vi "Main.vi"(11 "Module Admin":refnum<class "Delacor_lib_QMH_Cloneable Module Admin.lvclass">) -> ()   [LabVIEW 2023, in "EL72xxDMC_Drive.lvlib"]
doc: "This template is based off of the Queued Message Handler design pattern and the Queued Message Handler project template that ships with LabVIEW.\n\nThe main difference is that the queue is private to this module and communication between modules is performed via Broadcast and Request events.\n\nRequest events are wrapped in public API methods and are handled in the Event Handling Loop (EHL) of this VI. Any module can register for Broadcast events sent by this module. The EHL generates messages based on user interface actions.\n\nThe Message Handling Loop (MHL) processes messages generated by the EHL, or by other messages. The messages are string values, so new messages can be added easily to the Message Cases case structure in the MHL. Each message cluster can also provide an optional value for Message Data, which is a variant that can be converted to whatever message-specific data is required.\n_____\nBased on DQMH Project Template 7.0.1.1316."
uses:
  EL72xxDMC_Drive.lvlib
  <vilib>/Delacor/Delacor QMH/Libraries/Message Queue_class/Delacor_lib_QMH_Message Queue.lvclass
  Module Data--cluster.ctl
  <vilib>/Utility/miscctls.llb/LVPointTypeDef.ctl
  <vilib>/Delacor/Delacor QMH/Libraries/Message Queue_class/Delacor_lib_QMH_Enqueue Message (Single).vi
  Stop Argument--cluster.ctl
  <vilib>/Delacor/Delacor QMH/Libraries/Cloneable Module Admin_class/Delacor_lib_QMH_Cloneable Module Admin.lvclass
  ConnectToDrive Argument--cluster.ctl
  DisconnectFromDrive Argument--cluster.ctl
  EnableDrive Argument--cluster.ctl
  <userlib>/Beckhoff-LabVIEW-Interface/_DependsOn/Base/TypeResolver/Set TypeResolver.vi
  <userlib>/Beckhoff-LabVIEW-Interface/_DependsOn/Base/Write/Write Sync.vi
  DisableDrive Argument--cluster.ctl
panel:
  out "error out":errorcluster
  out "Status":string
  in  "Simulate EHL Error":bool
  in  "Simulate MHL Error":bool
  # "Other processes communicate with this Module via its Public API (wrappers for its Request Events).\n\nThis Module communicates with other processes via its Broadcast Events.\nAny process that wants to receive these messages can register for this module's Broadcast events."
  # "This template is for the DQMH framework. See the block diagram for more information on how to use this template."
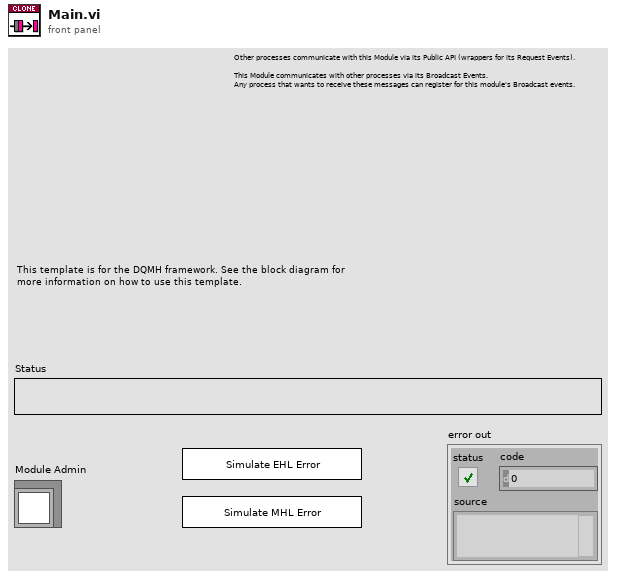
[diagram p1: front panel]
types:
  T1 = typedef "EL72xxDMC_Drive.lvlib/Request Events--cluster.ctl" = cluster{"Stop Module":refnum<user-event>, "Show Panel":refnum<user-event>, "Hide Panel":refnum<user-event>, "Show Diagram":refnum<user-event>, "Get Module Execution Status":refnum<user-event>, "ConnectToDrive":refnum<user-event>, "DisconnectFromDrive":refnum<user-event>, "EnableDrive":refnum<user-event>, "DisableDrive":refnum<user-event>}
  T2 = typedef "EL72xxDMC_Drive.lvlib/Module Data--cluster.ctl" = cluster{"Status":string}
  T3 = enum32{"invalid lock state", "Not Locked", "Locked (No Password)", "Password-protected"}
  T4 = typedef "EL72xxDMC_Drive.lvlib/Stop Argument--cluster.ctl" = cluster{"Module ID":i32, "Origin":string, "Exit via Stop Module Req?":bool, "Wait for Module to stop?":bool}
  T5 = typedef "EL72xxDMC_Drive.lvlib/ConnectToDrive Argument--cluster.ctl" = cluster{"Module ID":i32, "Pathway":string}
  T6 = typedef "EL72xxDMC_Drive.lvlib/DisconnectFromDrive Argument--cluster.ctl" = cluster{"Module ID":i32, "Boolean":bool}
  T7 = typedef "EL72xxDMC_Drive.lvlib/EnableDrive Argument--cluster.ctl" = cluster{"Module ID":i32, "Boolean":bool}
  T8 = typedef "EL72xxDMC_Drive.lvlib/DisableDrive Argument--cluster.ctl" = cluster{"Module ID":i32, "Boolean":bool}
  T9 = typedef "LVPointTypeDef.ctl" = cluster{"Horizontal":i16, "Vertical":i16}
  T10 = enum32{"Invalid", "Standard", "Closed", "Hidden", "Minimized", "Maximized"}
  T11 = cluster{"FeedbackControl":cluster{"Enable latch extern on positive edge":bool, "Set counter":bool, "Enable latch extern on negative edge":bool}, "DriveControl":cluster{"Enable":bool, "Reset":bool}, "PositioningControl":cluster{"Execute":bool, "Emergency stop":bool}, "Set counter value":i32, "Target position":i32, "Target velocity":i16, "Start type":u16, "Target acceleration":u16, "Target deceleration":u16}
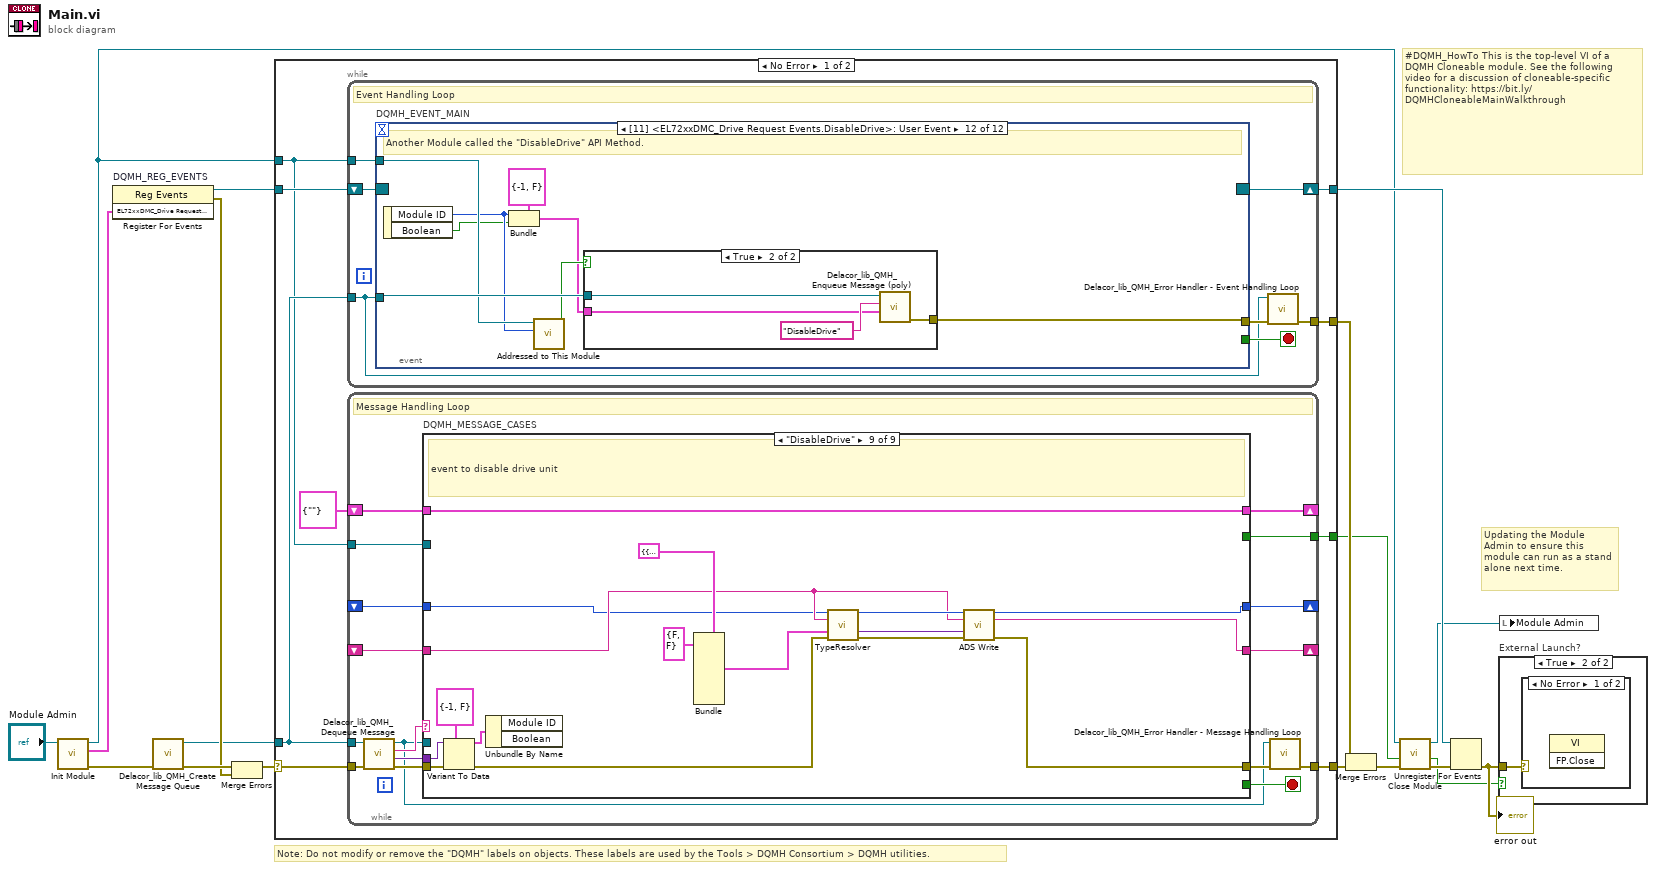
[diagram p0: block diagram]
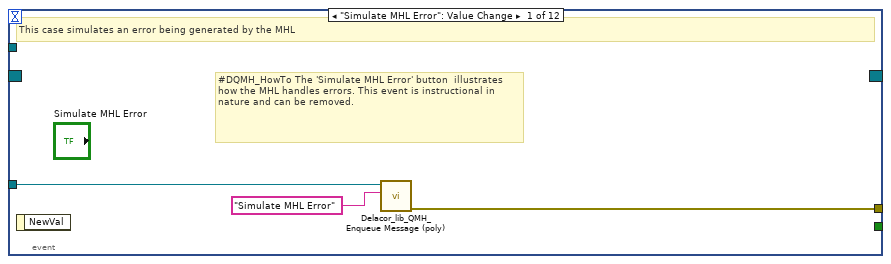
[diagram p2: hidden frame]
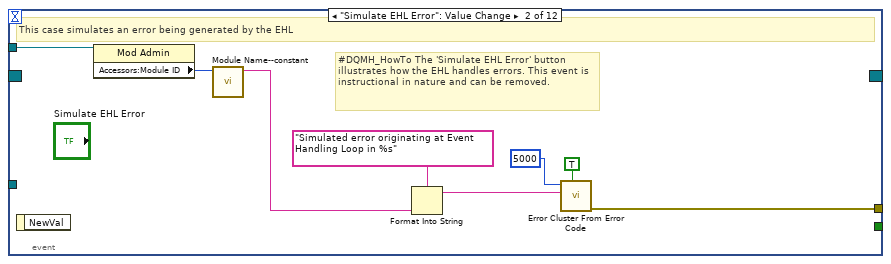
[diagram p3: hidden frame]
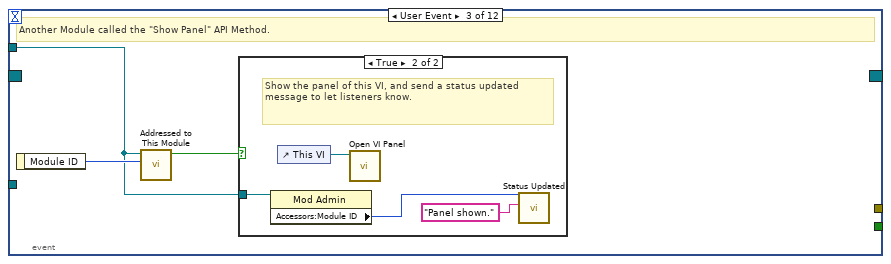
[diagram p4: hidden frame]
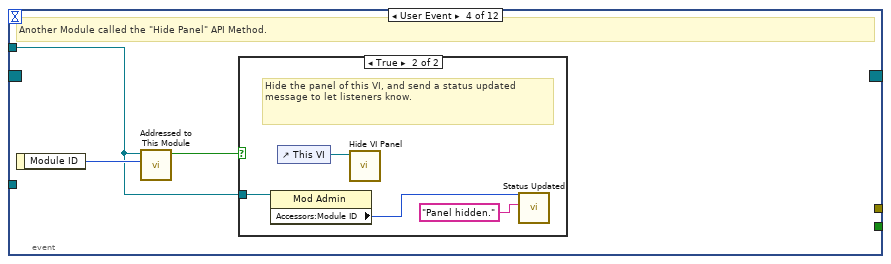
[diagram p6: hidden frame]
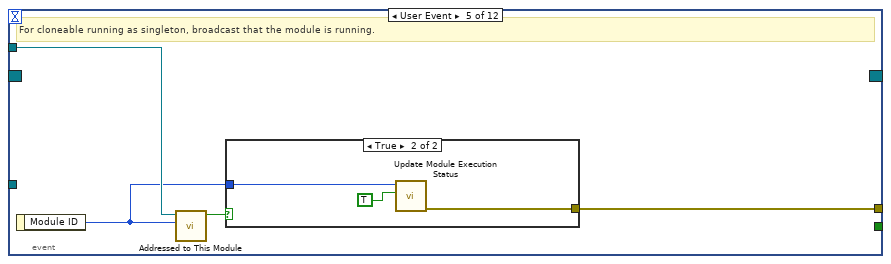
[diagram p8: hidden frame]
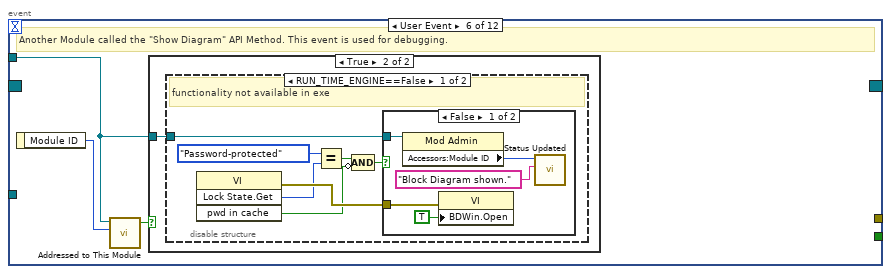
[diagram p10: hidden frame]
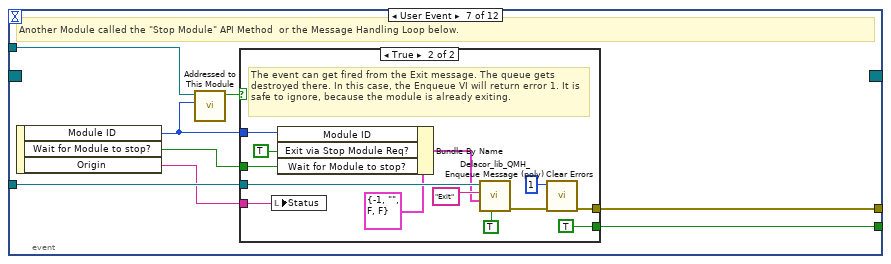
[diagram p14: hidden frame]
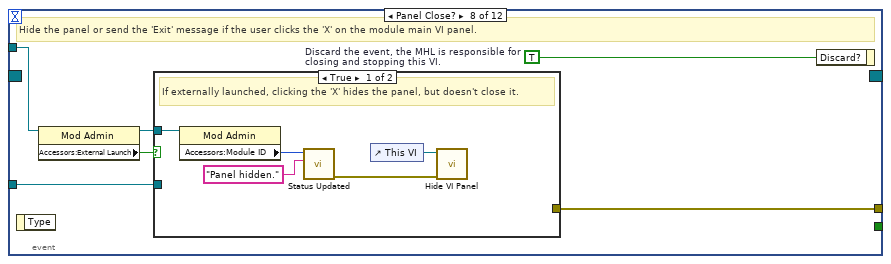
[diagram p16: hidden frame]
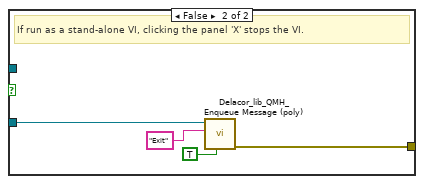
[diagram p17: hidden frame]
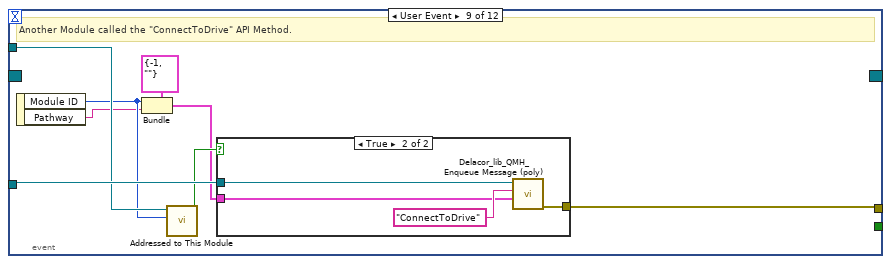
[diagram p18: hidden frame]
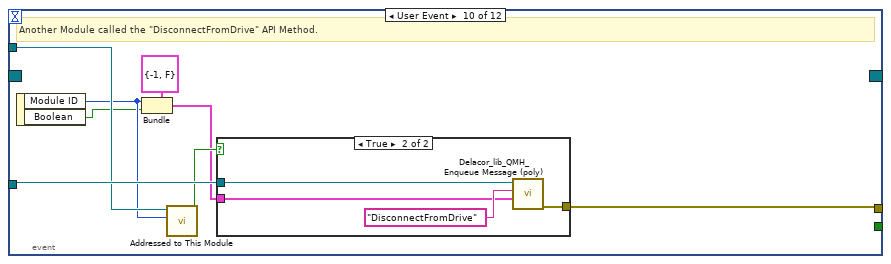
[diagram p20: hidden frame]
diagram:
  # "#DQMH_HowTo This is the top-level VI of a DQMH Cloneable module. See the following video for a discussion of cloneable-specific functionality: https://bit.ly/DQMHCloneableMainWalkthrough"
  # "Note: Do not modify or remove the \"DQMH\" labels on objects. These labels are used by the Tools > DQMH Consortium > DQMH utilities."
  # "Updating the Module Admin to ensure this module can run as a stand alone next time."
  n1 = call "Init Module.vi"("Cloneable Module Admin in"="Module Admin") -> ("error out"=w15:errorcluster, "EL72xxDMC_Drive Request Events"=w7:T1, "Cloneable Module Admin out"=w4:refnum<class "Delacor_lib_QMH_Cloneable Module Admin.lvclass">)  [unwired: 8 in]
  n2 = register-events "DQMH_REG_EVENTS"(w7) -> (reference out=w8:refnum<event-registration>, error out=w10:errorcluster)  [unwired: 2 in]
  n3 = call <vilib>:"Delacor_lib_QMH_Create Message Queue.vi"("error in"=w15) -> ("error out"=w12:errorcluster, "Message Queue"=w6:refnum<class "Delacor_lib_QMH_Message Queue.lvclass">)  [unwired: 9 in]
  n4 = Merge Errors(w12, w10) -> (w11:errorcluster)
  n5 = case shown="No Error" w11 {
    selector: w11 -> [w25 w338]
    tunnel: [w27 w337] -> w16
    tunnel: [w24 w336] -> w9
    tunnel: w8 -> [w22 w336]
    tunnel: w6 -> [w21 w329]
    tunnel: [w26 _] -> w17
    tunnel: w4 -> [w20 w332]
    tunnel: [w19 _] -> w2
    frame No Error {
      n6 = while {
        tunnel: w21 -> [w28]
        shift-right: [w31] -> w24
        shift-left: w22 -> [w32]
        tunnel: [w33] -> w26
        tunnel: w20 -> [w29]
        stop <- w30 stop-if-true
        # "Event Handling Loop"
        n7 = event "DQMH_EVENT_MAIN" shown="[11] <EL72xxDMC_Drive Request Events.DisableDrive>: User Event" {
          selector: w32 -> [_ _ _ _ _ _ _ _ _ _ _ _]
          dyn-events: [_ _ _ _ _ _ _ _ _ _ _ _] -> w31
          timeout: _ -> [_ _ _ _ _ _ _ _ _ _ _ _]
          tunnel: [_ _ _ _ _ _ w86 _ _ _ _ _] -> w30
          tunnel: w28 -> [w36 _ _ _ _ _ w89 w106 w126 w138 w150 w162]
          tunnel: [w37 w45 _ _ w63 _ w90 w109 w119 w131 w143 w155] -> w34
          tunnel: w29 -> [_ w44 w46 w53 w61 w67 w88 w107 w124 w136 w148 w160]
          event "Simulate MHL Error": Value Change {
            # "#DQMH_HowTo The 'Simulate MHL Error' button  illustrates how the MHL handles errors. This event is instructional in nature and can be removed."
            # "This case simulates an error being generated by the MHL"
            n8 = event-data() -> ()  [unwired: 1 in, 1 out]
            n9 = call-poly <vilib>:"Delacor_lib_QMH_Enqueue Message (poly).vi"("Message"="Simulate MHL Error", "Message Queue in"=w36) -> ("error out"=w37:errorcluster)  [unwired: 8 in, 1 out]
          }
          event "Simulate EHL Error": Value Change {
            # "#DQMH_HowTo The 'Simulate EHL Error' button  illustrates how the EHL handles errors. This event is instructional in nature and can be removed."
            # "This case simulates an error being generated by the EHL"
            n10 = event-data() -> ()  [unwired: 1 in, 1 out]
            n11 = property on="Property Node" class="Mod Admin"(reference=w44) -> ("Accessors:Module ID"=w43:i32)  [unwired: 1 in, 2 out]
            n12 = call "Module Name--constant.vi"("Module ID"=w43) -> ("Module Name"=w38:string)  [unwired: 10 in]
            n13 = Format Into String(format string="Simulated error originating at Event Handling Loop in %s", w38) -> (resulting string=w41:string)  [unwired: 2 in, 1 out]
            n14 = call <vilib>:"Error Cluster From Error Code.vi"("show call chain? (False)"=TRUE, "error message (\"\")"=w41, "error code (0)"=5000) -> ("error out"=w45:errorcluster)  [unwired: 6 in]
          }
          event User Event {
            # "Another Module called the \"Show Panel\" API Method."
            n15 = event-data() -> ("Module ID"=w47:i32)  [unwired: 1 in]
            n16 = call "Addressed to This Module.vi"("Module ID from Argument"=w47, "Module Admin"=w46) -> ("Addressed to this instance?"=w48:bool)  [unwired: 8 in, 1 out]
            n17 = case shown="True" w48 {
              tunnel: w46 -> [_ w50]
              frame False {
              }
              frame True {
                # "Show the panel of this VI, and send a status updated message to let listeners know."
                n18 = property on="Property Node" class="Mod Admin"(reference=w50) -> ("Accessors:Module ID"=w49:i32)  [unwired: 1 in, 2 out]
                n19 = control-ref of="This VI"() -> (w52:refnum<vi>)
                n20 = call "Open VI Panel.vi"("VI"=w52) -> ()  [unwired: 10 in, 1 out]
                n21 = call "Status Updated.vi"("Status"="Panel shown." ("format string"), "Module ID"=w49) -> ()  [unwired: 9 in, 1 out]
              }
            }
          }
          event User Event {
            # "Another Module called the \"Hide Panel\" API Method."
            n22 = event-data() -> ("Module ID"=w54:i32)  [unwired: 1 in]
            n23 = call "Addressed to This Module.vi"("Module ID from Argument"=w54, "Module Admin"=w53) -> ("Addressed to this instance?"=w55:bool)  [unwired: 8 in, 1 out]
            n24 = case shown="True" w55 {
              tunnel: w53 -> [_ w57]
              frame False {
              }
              frame True {
                # "Hide the panel of this VI, and send a status updated message to let listeners know."
                n25 = property on="Property Node" class="Mod Admin"(reference=w57) -> ("Accessors:Module ID"=w56:i32)  [unwired: 1 in, 2 out]
                n26 = control-ref of="This VI"() -> (w59:refnum<vi>)
                n27 = call "Hide VI Panel.vi"("VI"=w59) -> ()  [unwired: 10 in, 1 out]
                n28 = call "Status Updated.vi"("Status"="Panel hidden." ("format string"), "Module ID"=w56) -> ()  [unwired: 9 in, 1 out]
              }
            }
          }
          event User Event {
            # "For cloneable running as singleton, broadcast that the module is running."
            n29 = event-data() -> ("Module ID"=w60:i32)  [unwired: 1 in]
            n30 = call "Addressed to This Module.vi"("Module ID from Argument"=w60, "Module Admin"=w61) -> ("Addressed to this instance?"=w62:bool)  [unwired: 8 in, 1 out]
            n31 = case shown="True" w62 {
              tunnel: [_ w66] -> w63
              tunnel: w60 -> [_ w65]
              frame False {
              }
              frame True {
                n32 = call "Update Module Execution Status.vi"("Running?"=TRUE, "Module ID"=w65) -> ("error out"=w66:errorcluster)  [unwired: 9 in]
              }
            }
          }
          event User Event {
            # "Another Module called the \"Show Diagram\" API Method. This event is used for debugging."
            n33 = event-data() -> ("Module ID"=w68:i32)  [unwired: 1 in]
            n34 = call "Addressed to This Module.vi"("Module ID from Argument"=w68, "Module Admin"=w67) -> ("Addressed to this instance?"=w69:bool)  [unwired: 8 in, 1 out]
            n35 = case shown="True" w69 {
              tunnel: w67 -> [_ w70]
              frame False {
              }
              frame True {
                n36 = disable-structure shown="RUN_TIME_ENGINE==False" {
                  disable-tunnel: w70 -> [w71 _]
                  frame condition #0 (active) {
                    # "functionality not available in exe"
                    n37 = invoke on="Invoke Node" class="VI" method="Lock State.Get"() -> (error out=w77:errorcluster, "Get Lock State"=w76:T3, "pwd in cache"=w73:bool)  [unwired: 4 in, 1 out]
                    n38 = Equal?(x=T3."Password-protected", y=w76) -> (x = y?=w74:bool)
                    n39 = Compound Arithmetic op=AND(w74, invert w73) -> (w72:bool)
                    n40 = case shown="False" w72 {
                      tunnel: w77 -> [w82 _]
                      tunnel: w71 -> [w79 _]
                      frame False {
                        n41 = property on="Property Node" class="Mod Admin"(reference=w79) -> ("Accessors:Module ID"=w78:i32)  [unwired: 1 in, 2 out]
                        n42 = property on="Property Node" class="VI"(error in=w82, "BDWin.Open"=TRUE ("Block Diagram Window:Open")) -> ()  [unwired: 1 in, 2 out]
                        n43 = call "Status Updated.vi"("Status"="Block Diagram shown." ("format string"), "Module ID"=w78) -> ()  [unwired: 9 in, 1 out]
                      }
                      frame True {
                        # "Password-protected VI, and the password is not in the cache. Do not show the diagram."
                      }
                    }
                  }
                  frame condition #1 {
                  }
                }
              }
            }
          }
          event User Event {
            # "Another Module called the \"Stop Module\" API Method  or the Message Handling Loop below."
            n44 = event-data() -> ("Module ID"=w84:i32, "Wait for Module to stop?"=w85:bool, "Origin"=w83:string)  [unwired: 1 in]
            n45 = call "Addressed to This Module.vi"("Module ID from Argument"=w84, "Module Admin"=w88) -> ("Addressed to this instance?"=w87:bool)  [unwired: 8 in, 1 out]
            n46 = case shown="True" w87 {
              tunnel: [_ w102] -> w90
              tunnel: w89 -> [_ w98]
              tunnel: [_ TRUE] -> w86
              tunnel: w85 -> [_ w93]
              tunnel: w84 -> [_ w95]
              tunnel: w83 -> [_ w91]
              frame False {
              }
              frame True {
                # "The event can get fired from the Exit message. The queue gets destroyed there. In this case, the Enqueue VI will return error 1. It is safe to ignore, because the module is already exiting."
                n47 = local write "Status"(w91) -> ()
                n48 = Bundle By Name(cluster=T4 {"Module ID"=-1, "Origin"="", "Exit via Stop Module Req?"=FALSE, "Wait for Module to stop?"=FALSE} ("Stop Argument"), "Module ID"=w95, "Exit via Stop Module Req?"=TRUE, "Wait for Module to stop?"=w93) -> (w92:T4)
                n49 = call-poly <vilib>:"Delacor_lib_QMH_Enqueue Message (poly).vi"("Priority Message? (F)"=TRUE, "Message Data"=w92, "Message"="Exit", "Message Queue in"=w98) -> ("error out"=w103:errorcluster)  [unwired: 6 in, 1 out]
                n50 = call <vilib>:"Clear Errors.vi"("error in (no error)"=w103, "specific error code to clear (0: all)"=1) -> ("error out"=w102:errorcluster)  [unwired: 4 in, 1 out]
              }
            }
          }
          event Panel Close? {
            w108 = TRUE  # Discard the event, the MHL is responsible for closing and stopping this VI.
            # "Hide the panel or send the 'Exit' message if the user clicks the 'X' on the module main VI panel."
            n51 = event-data() -> ()  [unwired: 1 in, 1 out]
            n52 = property on="Property Node" class="Mod Admin"(reference=w107) -> (reference out=w104:refnum<class "Delacor_lib_QMH_Cloneable Module Admin.lvclass">, "Accessors:External Launch"=w105:bool)  [unwired: 1 in, 1 out]
            n53 = case shown="True" w105 {
              tunnel: w106 -> [_ w117]
              tunnel: [_ w118] -> w109
              tunnel: w104 -> [w112 _]
              frame True {
                # "If externally launched, clicking the 'X' hides the panel, but doesn't close it."
                n54 = property on="Property Node" class="Mod Admin"(reference=w112) -> ("Accessors:Module ID"=w111:i32)  [unwired: 1 in, 2 out]
                n55 = call "Status Updated.vi"("Status"="Panel hidden." ("format string"), "Module ID"=w111) -> ("error out"=w110:errorcluster)  [unwired: 9 in]
                n56 = control-ref of="This VI"() -> (w114:refnum<vi>)
                n57 = call "Hide VI Panel.vi"("error in"=w110, "VI"=w114) -> ()  [unwired: 9 in, 1 out]
              }
              frame False {
                # "If run as a stand-alone VI, clicking the panel 'X' stops the VI."
                n58 = call-poly <vilib>:"Delacor_lib_QMH_Enqueue Message (poly).vi"("Priority Message? (F)"=TRUE, "Message"="Exit", "Message Queue in"=w117) -> ("error out"=w118:errorcluster)  [unwired: 7 in, 1 out]
              }
            }
            n59 = event-data ("Event Filter Node")("Discard?"=w108) -> ()  [unwired: 1 in, 1 out]
          }
          event User Event {
            # "Another Module called the \"ConnectToDrive\" API Method."
            n60 = event-data() -> ("Module ID"=w121:i32, "Pathway"=w120:string)  [unwired: 1 in]
            n61 = Bundle(cluster=T5 {"Module ID"=-1, "Pathway"=""} ("ConnectToDrive Argument"), "Module ID"=w121, "Pathway"=w120) -> (w122:T5)
            n62 = call "Addressed to This Module.vi"("Module ID from Argument"=w121, "Module Admin"=w124) -> ("Addressed to this instance?"=w125:bool)  [unwired: 8 in, 1 out]
            n63 = case shown="True" w125 {
              tunnel: w126 -> [_ w130]
              tunnel: w122 -> [_ w128]
              tunnel: [_ w127] -> w119
              frame False {
              }
              frame True {
                n64 = call-poly <vilib>:"Delacor_lib_QMH_Enqueue Message (poly).vi"("Message Data"=w128, "Message"="ConnectToDrive", "Message Queue in"=w130) -> ("error out"=w127:errorcluster)  [unwired: 7 in, 1 out]
              }
            }
          }
          event User Event {
            # "Another Module called the \"DisconnectFromDrive\" API Method."
            n65 = event-data() -> ("Module ID"=w133:i32, "Boolean"=w132:bool)  [unwired: 1 in]
            n66 = Bundle(cluster=T6 {"Module ID"=-1, "Boolean"=FALSE} ("DisconnectFromDrive Argument"), "Module ID"=w133, "Boolean"=w132) -> (w134:T6)
            n67 = call "Addressed to This Module.vi"("Module ID from Argument"=w133, "Module Admin"=w136) -> ("Addressed to this instance?"=w137:bool)  [unwired: 8 in, 1 out]
            n68 = case shown="True" w137 {
              tunnel: w138 -> [_ w142]
              tunnel: w134 -> [_ w140]
              tunnel: [_ w139] -> w131
              frame False {
              }
              frame True {
                n69 = call-poly <vilib>:"Delacor_lib_QMH_Enqueue Message (poly).vi"("Message Data"=w140, "Message"="DisconnectFromDrive", "Message Queue in"=w142) -> ("error out"=w139:errorcluster)  [unwired: 7 in, 1 out]
              }
            }
          }
          event User Event {
            # "Another Module called the \"EnableDrive\" API Method."
            n70 = event-data() -> ("Module ID"=w145:i32, "Boolean"=w144:bool)  [unwired: 1 in]
            n71 = Bundle(cluster=T7 {"Module ID"=-1, "Boolean"=FALSE} ("EnableDrive Argument"), "Module ID"=w145, "Boolean"=w144) -> (w146:T7)
            n72 = call "Addressed to This Module.vi"("Module ID from Argument"=w145, "Module Admin"=w148) -> ("Addressed to this instance?"=w149:bool)  [unwired: 8 in, 1 out]
            n73 = case shown="True" w149 {
              tunnel: w150 -> [_ w154]
              tunnel: w146 -> [_ w152]
              tunnel: [_ w151] -> w143
              frame False {
              }
              frame True {
                n74 = call-poly <vilib>:"Delacor_lib_QMH_Enqueue Message (poly).vi"("Message Data"=w152, "Message"="EnableDrive", "Message Queue in"=w154) -> ("error out"=w151:errorcluster)  [unwired: 7 in, 1 out]
              }
            }
          }
          event User Event {
            # "Another Module called the \"DisableDrive\" API Method."
            n75 = event-data() -> ("Module ID"=w157:i32, "Boolean"=w156:bool)  [unwired: 1 in]
            n76 = Bundle(cluster=T8 {"Module ID"=-1, "Boolean"=FALSE} ("DisableDrive Argument"), "Module ID"=w157, "Boolean"=w156) -> (w158:T8)
            n77 = call "Addressed to This Module.vi"("Module ID from Argument"=w157, "Module Admin"=w160) -> ("Addressed to this instance?"=w161:bool)  [unwired: 8 in, 1 out]
            n78 = case shown="True" w161 {
              tunnel: w162 -> [_ w166]
              tunnel: w158 -> [_ w164]
              tunnel: [_ w163] -> w155
              frame False {
              }
              frame True {
                n79 = call-poly <vilib>:"Delacor_lib_QMH_Enqueue Message (poly).vi"("Message Data"=w164, "Message"="DisableDrive", "Message Queue in"=w166) -> ("error out"=w163:errorcluster)  [unwired: 7 in, 1 out]
              }
            }
          }
        }
        n80 = call-dynamic "Delacor_lib_QMH_Error Handler - Event Handling Loop.vi"("error in"=w34, "Message Queue in"=w28) -> ("dup error in"=w33:errorcluster)  [unwired: 8 in, 1 out]
      }
      n81 = while {
        tunnel: w21 -> [w171]
        shift-right: [w178] -> _
        shift-left: T2 {"Status"=""} ("Data Cluster") -> [w179]
        tunnel: w25 -> [w182]
        tunnel: [w180] -> w27
        tunnel: w20 -> [w173]
        tunnel: [w172] -> w19
        shift-right: [w170] -> _
        shift-left: _ -> [w167]
        shift-right: [w169] -> _
        shift-left: _ -> [w168]
        stop <- w177 stop-if-true
        # "Message Handling Loop"
        n82 = call-dynamic "Delacor_lib_QMH_Dequeue Message.vi"("error in"=w182, "Message Queue in"=w171) -> ("error out"=w181:errorcluster, "Message Data"=w175:variant, "Message"=w176:string, "Message Queue out"=w174:refnum<class "Delacor_lib_QMH_Message Queue.lvclass">)  [unwired: 6 in]
        n83 = case "DQMH_MESSAGE_CASES" shown="\"DisableDrive\"" w176 {
          selector: w176 -> [_ _ _ _ _ w274 _ _ _]
          tunnel: w174 -> [_ _ w223 _ w264 _ _ _ _]
          tunnel: w181 -> [w204 w218 w232 w251 w270 w283 w294 w311 w328]
          tunnel: [w202 w211 w228 w250 w265 w284 w287 w302 w312] -> w183
          tunnel: w179 -> [w195 w217 w227 w248 w263 w281 w293 w310 w327]
          tunnel: [w194 w217 w227 w248 w263 w281 w293 w310 w327] -> w178
          tunnel: [_ _ _ _ w262 _ _ _ _] -> w177
          tunnel: w175 -> [_ w216 w226 _ w260 _ w292 w309 w326]
          tunnel: w173 -> [w189 _ w225 w246 w255 w280 _ _ _]
          tunnel: [_ _ _ _ w258 _ _ _ _] -> w172
          tunnel: [u32 0 ("Handle") w210 u32 0 ("Handle") u32 0 ("Handle") u32 0 ("Handle") w271 u32 0 ("Handle") w299 w315] -> w170
          tunnel: ["" ("ReadGrpSymbols") w207 "" ("ReadGrpSymbols") "" ("ReadGrpSymbols") "" ("ReadGrpSymbols") w272 "" ("ReadGrpSymbols") w298 w314] -> w169
          tunnel: w168 -> [_ _ _ _ _ w272 _ w300 w317]
          tunnel: w167 -> [_ _ _ _ _ w271 w289 w306 w316]
          frame "Initialize" {
            w186 = "Initial Message" ("Initial Message")
            # "#CodeNeeded - Initialize the appearance of the front panel."
            # "#CodeNeeded - Initialize your state data here."
            # "Initialize - Any operation that needs to be done before the module can receive messages. Synchronize Caller Events.vi will inform Start Module.vi that the module has launched and is ready to receive messages. Module Did Init.vi will broadcast that the module initialized."
            n84 = call "Synchronize Caller Events.vi"("error in"=w204, "Module Admin"=w189) -> ("error out"=w203:errorcluster, "Module Admin out"=w188:refnum<class "Delacor_lib_QMH_Cloneable Module Admin.lvclass">)  [unwired: 8 in]
            n85 = property on="Property Node" class="Mod Admin"(reference=w188) -> ("Accessors:Module ID"=w191:i32, "Accessors:External Launch"=w190:bool)  [unwired: 1 in, 2 out]
            n86 = call "Module Name--constant.vi"("Module ID"=w191) -> ("Module Name"=w199:string)  [unwired: 10 in]
            n87 = property on="Property Node" class="VI"("Front Panel.Title"=w199) -> (reference out=w201:refnum<vi>, error out=w206:errorcluster)  [unwired: 2 in]
            n88 = Select(t=T10."Hidden" ("State"), s=w190, f=T10."Standard" ("State")) -> (s? t:f=w196:T10)
            n89 = invoke on="Invoke Node" class="VI" method="FP.Open"(reference=w201, error in=w206, "State"=w196) -> (reference out=w200:refnum<vi>, error out=w205:errorcluster)  [unwired: 2 in, 3 out]
            n90 = call "Module Name--constant.vi"("Module ID"=w191) -> ("Module Name"=w192:string)  [unwired: 10 in]
            n91 = Bundle By Name(cluster=w195, "Status"=w186) -> (w194:T2)
            n92 = invoke on="Invoke Node" class="VI" method="FP.Center"(reference=w200, error in=w205) -> ()  [unwired: 1 in, 3 out]
            n93 = property on="Pane" class="Pane"("Origin"=T9 {"Horizontal"=0, "Vertical"=0}) -> ()  [unwired: 2 in, 2 out]
            n94 = call "Module Did Init.vi"("error in"=w203, "Initialized?"=TRUE, "Origin"=w192, "Module ID"=w191) -> ("error out"=w202:errorcluster)  [unwired: 7 in]
            "Status" <- w186
          }
          frame "ConnectToDrive" {
            # "event to create a connection to a drive terminal"
            n95 = Variant To Data(error in=w218, type=T5 {"Module ID"=-1, "Pathway"=""} ("ConnectToDrive Argument"), Variant=w216) -> (data=w214:T5, error out=w212:errorcluster)
            n96 = Unbundle By Name(w214) -> ("Pathway"=w213:string)  [unwired: 1 out]
            n97 = call <userlib>:"Init.vi"("XMLDescription"=w213, "error in (no error)"=w212) -> ("Handle"=w210:u32, "WriteGrpSymbols"=w209:string[], "error out"=w211:errorcluster)  [unwired: 9 in, 2 out]
            n98 = Index Array(array=w209, index=0) -> (element=w207:string)
          }
          frame "Error" {
            # "#CodeRecommended - If the module is running in standalone mode (External Launch = FALSE), this code will pop up an error dialog and call the 'Exit' message if an error occurs. Add more fine-grained error management here."
            # "Error - Check the error message data and respond accordingly. This message is sent by the \"Error Handler\" VIs at the end of each loop in this application."
            n99 = property on="Property Node" class="Mod Admin"(reference=w225) -> ("Accessors:External Launch"=w224:bool, "Accessors:Module ID"=w222:i32)  [unwired: 1 in, 2 out]
            n100 = Variant To Data(error in=w232, type=errorcluster {"status"=FALSE, "code"=0, "source"=""} ("error constant"), Variant=w226) -> (data=w221:errorcluster, error out=w230:errorcluster)
            n101 = local write "error out"(w221) -> ()
            n102 = call "Error Reported.vi"("Error"=w221, "Module ID"=w222) -> ()  [unwired: 9 in, 1 out]
            n103 = case shown="False" w224 {
              tunnel: [w237 _] -> w229
              tunnel: w223 -> [w235 _]
              tunnel: w221 -> [w236 _]
              frame False {
                n104 = disable-structure shown="Default" {
                  disable-tunnel: w236 -> [w238 _]
                  frame condition #0 (active) {
                    # "If the module is running standalone, then pop up an error dialog and call the \"Exit\" message."
                    n105 = call <vilib>:"Simple Error Handler.vi"("error in (no error)"=w238) -> ()  [unwired: 4 in, 5 out]
                  }
                  frame condition #1 {
                    # "To prevent the Simple Error Handler VI from being loaded (e.g. when deploying to a Real-Time target), add the Conditional Disable Symbol \"DQMH_Disable_SEH\" to your project and set it to TRUE."
                  }
                }
                n106 = call-poly <vilib>:"Delacor_lib_QMH_Enqueue Message (poly).vi"("Priority Message? (F)"=TRUE, "Message"="Exit", "Message Queue in"=w235) -> ("error out"=w237:errorcluster)  [unwired: 7 in, 1 out]
              }
              frame True {
                # "If the module was launched externally, calling the Error Reported broadcast VI is the only action performed by the \"Error\" message. The module's caller can then process the error appropriately."
              }
            }
            n107 = Merge Errors(w230, w229) -> (w228:errorcluster)
          }
          frame "Simulate MHL Error" {
            # "#DQMH_HowTo The 'Simulate MHL Error' button  illustrates how the MHL handles errors. This event is instructional in nature and can be removed."
            # "Simulate an error occurring at the MHL"
            n108 = property on="Property Node" class="Mod Admin"(reference=w246) -> ("Accessors:Module ID"=w247:i32)  [unwired: 1 in, 2 out]
            n109 = call "Module Name--constant.vi"("Module ID"=w247) -> ("Module Name"=w242:string)  [unwired: 10 in]
            n110 = Format Into String(format string="Simulated error originating at Message Handling Loop in %s", w242) -> (resulting string=w243:string)  [unwired: 2 in, 1 out]
            n111 = call <vilib>:"Error Cluster From Error Code.vi"("show call chain? (False)"=TRUE, "error message (\"\")"=w243, "error code (0)"=5001) -> ("error out"=w249:errorcluster)  [unwired: 6 in]
            n112 = Merge Errors(w251, w249) -> (w250:errorcluster)
          }
          frame "Exit" {
            w261 = 91  # 91: not all Exit messages will have an argument
            w262 = TRUE  # Stop the VI
            # "Release the message queue reference"
            # "#CodeNeeded - Add any required cleanup code here."
            # "Exit - Exit the application."
            n113 = Variant To Data(error in=w270, type=T4 {"Module ID"=-1, "Origin"="", "Exit via Stop Module Req?"=FALSE, "Wait for Module to stop?"=FALSE} ("Stop Argument"), Variant=w260) -> (data=w257:T4, error out=w266:errorcluster)
            n114 = call <vilib>:"Clear Errors.vi"("error in (no error)"=w266, "specific error code to clear (0: all)"=w261) -> ("error out"=w269:errorcluster)  [unwired: 4 in, 1 out]
            n115 = property on="Property Node" class="Mod Admin"(reference=w255) -> ("Accessors:Module ID"=w254:i32)  [unwired: 1 in, 2 out]
            n116 = control-ref of="This VI"() -> (w256:refnum<vi>)
            n117 = call-dynamic "Delacor_lib_QMH_Release Message Queue.vi"("error in"=w269, "Message Queue"=w264) -> ("error out"=w268:errorcluster)  [unwired: 9 in]
            n118 = call "Handle Exit.vi"("Stop Argument"=w257, "Module Admin in"=w255, "VI reference"=w256) -> ("error out"=w267:errorcluster, "Wait for Stop?"=w258:bool)  [unwired: 7 in]
            n119 = Merge Errors(w268, w267) -> (w265:errorcluster)
            n120 = call "Error Reported.vi"("Error"=w265, "Module ID"=w254) -> ()  [unwired: 9 in, 1 out]
          }
          frame Default {
            # "'Default' case only runs if there is a message that isn't defined in any of the other cases.  Output a programming error."
            n121 = property on="Property Node" class="Mod Admin"(reference=w280) -> ("Accessors:Module ID"=w279:i32)  [unwired: 1 in, 2 out]
            n122 = call "Module Name--constant.vi"("Module ID"=w279) -> ("Module Name"=w273:string)  [unwired: 10 in]
            n123 = Format Into String(format string="The invalid message string \"%s\" was received in the Message Handling Loop for module \"%s\".", w274, w273) -> (resulting string=w276:string)  [unwired: 2 in, 1 out]
            n124 = call <vilib>:"Error Cluster From Error Code.vi"("show call chain? (False)"=TRUE, "error message (\"\")"=w276, "error code (0)"=1) -> ("error out"=w282:errorcluster)  [unwired: 6 in]
            n125 = Merge Errors(w283, w282) -> (w284:errorcluster)
          }
          frame "DisconnectFromDrive" {
            # "event to disconnect from a drive temrinal"
            n126 = Variant To Data(error in=w294, type=T6 {"Module ID"=-1, "Boolean"=FALSE} ("DisconnectFromDrive Argument"), Variant=w292) -> (data=w290:T6, error out=w288:errorcluster)
            n127 = Unbundle By Name(w290) -> ()  [unwired: 2 out]
            n128 = call <userlib>:"Release.vi"("Handle"=w289, "error in (no error)"=w288) -> ("error out"=w287:errorcluster)  [unwired: 13 in]
          }
          frame "EnableDrive" {
            n129 = Variant To Data(error in=w311, type=T7 {"Module ID"=-1, "Boolean"=FALSE} ("EnableDrive Argument"), Variant=w309) -> (data=w307:T7, error out=w305:errorcluster)
            n130 = Unbundle By Name(w307) -> ()  [unwired: 2 out]
            n131 = Bundle(cluster=T11 {"FeedbackControl"={"Enable latch extern on positive edge"=FALSE, "Set counter"=FALSE, "Enable latch extern on negative edge"=FALSE}, "DriveControl"={"Enable"=FALSE, "Reset"=FALSE}, "PositioningControl"={"Execute"=FALSE, "Emergency stop"=FALSE}, "Set counter value"=0, "Target position"=0, "Target velocity"=0, "Start type"=0, "Target acceleration"=0, "Target deceleration"=0} ("DMC_5CE8729A"), "DriveControl"=cluster{"Enable":bool, "Reset":bool} {"Enable"=TRUE, "Reset"=FALSE}) -> (w295:T11)  [unwired: 8 in]
            n132 = call-poly <userlib>:"TypeResolver.vi"("Handle"=w306, "SymbolName"=w300, "WData"=w295, "error in"=w305) -> ("Handle"=w304:u32, "ADSWData"=w301:variant, "error out"=w303:errorcluster)  [unwired: 8 in, 1 out]
            n133 = call-poly <userlib>:"ADS Write.vi"("Handle"=w304, "SymbolName"=w300, "Ads Write Data"=w301, "error in (no error)"=w303) -> ("Handle"=w299:u32, "SymbolName"=w298:string, "error out"=w302:errorcluster)  [unwired: 8 in, 1 out]
          }
          frame "DisableDrive" {
            # "event to disable drive unit"
            n134 = Variant To Data(error in=w328, type=T8 {"Module ID"=-1, "Boolean"=FALSE} ("DisableDrive Argument"), Variant=w326) -> (data=w324:T8, error out=w313:errorcluster)
            n135 = Unbundle By Name(w324) -> ()  [unwired: 2 out]
            n136 = Bundle(cluster=T11 {"FeedbackControl"={"Enable latch extern on positive edge"=FALSE, "Set counter"=FALSE, "Enable latch extern on negative edge"=FALSE}, "DriveControl"={"Enable"=FALSE, "Reset"=FALSE}, "PositioningControl"={"Execute"=FALSE, "Emergency stop"=FALSE}, "Set counter value"=0, "Target position"=0, "Target velocity"=0, "Start type"=0, "Target acceleration"=0, "Target deceleration"=0} ("DMC_5CE8729A"), "DriveControl"=cluster{"Enable":bool, "Reset":bool} {"Enable"=FALSE, "Reset"=FALSE}) -> (w323:T11)  [unwired: 8 in]
            n137 = call-poly <userlib>:"TypeResolver.vi"("Handle"=w316, "SymbolName"=w317, "WData"=w323, "error in"=w313) -> ("Handle"=w320:u32, "ADSWData"=w322:variant, "error out"=w321:errorcluster)  [unwired: 8 in, 1 out]
            n138 = call-poly <userlib>:"ADS Write.vi"("Handle"=w320, "SymbolName"=w317, "Ads Write Data"=w322, "error in (no error)"=w321) -> ("Handle"=w315:u32, "SymbolName"=w314:string, "error out"=w312:errorcluster)  [unwired: 8 in, 1 out]
          }
        }
        n139 = call-dynamic "Delacor_lib_QMH_Error Handler - Message Handling Loop.vi"("error in"=w183, "Message Queue in"=w174) -> ("dup error in"=w180:errorcluster)  [unwired: 8 in, 1 out]
      }
    }
    frame Error {
      n140 = call "Synchronize Caller Events.vi"("Module Admin"=w332) -> ("Module Admin out"=w331:refnum<class "Delacor_lib_QMH_Cloneable Module Admin.lvclass">)  [unwired: 9 in, 1 out]
      n141 = property on="Property Node" class="Mod Admin"(reference=w331) -> ("Accessors:Module ID"=w330:i32)  [unwired: 1 in, 2 out]
      n142 = call-dynamic "Delacor_lib_QMH_Release Message Queue.vi"("error in"=w338, "Message Queue"=w329) -> ("error out"=w337:errorcluster)  [unwired: 9 in]
      n143 = call "Module Name--constant.vi"("Module ID"=w330) -> ("Module Name"=w335:string)  [unwired: 10 in]
      n144 = Format Into String(format string="An error occurred during initialization. %s is no longer running.", w335) -> (resulting string=w333:string)  [unwired: 2 in, 1 out]
      n145 = call "Error Reported.vi"("Additional Information"=w333, "Error"=w337, "Module ID"=w330) -> ()  [unwired: 8 in, 1 out]
    }
  }
  n146 = Merge Errors(w17, w16) -> (w18:errorcluster)
  n147 = call "Close Module.vi"("error in"=w18, "Wait for stop?"=w2, "Module Admin in"=w4) -> ("error out"=w14:errorcluster, "External Launch"=w1:bool, "Module Admin out"=w3:refnum<class "Delacor_lib_QMH_Cloneable Module Admin.lvclass">)  [unwired: 6 in]
  n148 = Unregister For Events(event registration refnum=w9, error in=w14) -> (error out=w13:errorcluster)
  "error out" <- w13
  n149 = case "External Launch?" shown="True" w1 {
    tunnel: w13 -> [_ w339]
    frame False {
    }
    frame True {
      n150 = case shown="No Error" w339 {
        frame No Error {
          n151 = invoke class="VI" method="FP.Close"() -> ()  [unwired: 3 in, 3 out]
        }
        frame Error {
          n152 = invoke class="VI" method="FP.Open"("Activate"=TRUE ("Activate?")) -> ()  [unwired: 4 in, 5 out]
        }
      }
    }
  }
  n153 = local write "Module Admin"(w3) -> ()
